vi "resetKeithley.vi"   [LabVIEW 2011, in "run.lvlib"]
uses:
  run.lvlib
  <instrlib>/Keithley 2600 Series/Keithley 2600 Series.lvlib
types:
  T1 = enum16{"Digital I/O", "TSP-Link", "LAN", "Blender", "Timer"}
  T2 = enum16{"Digital I/O", "TSP-Link", "LAN", "Blender", "Timer"}[]
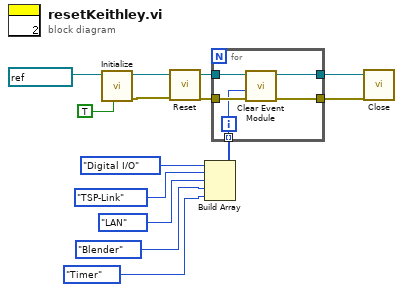
[diagram p0: block diagram]
diagram:
  n1 = call <instrlib>:"Initialize.vi"("Reset (True)"=TRUE, "VISA resource name"=refnum<visa-resource-name> "k2602a") -> ("error out"=w11:errorcluster, "VISA resource name out"=w12:refnum<visa-resource-name>)  [unwired: 8 in]
  n2 = call <instrlib>:"Reset.vi"("error in (no error)"=w11, "VISA resource name"=w12) -> ("error out"=w3:errorcluster, "VISA resource name out"=w5:refnum<visa-resource-name>)  [unwired: 8 in]
  n3 = Build Array(T1."Digital I/O" ("Event Module Type (Digital I/O)"), T1."TSP-Link" ("Event Module Type (Digital I/O)"), T1."LAN" ("Event Module Type (Digital I/O)"), T1."Blender" ("Event Module Type (Digital I/O)"), T1."Timer" ("Event Module Type (Digital I/O)")) -> (w1:T2)
  n4 = for {
    tunnel: w5 -> [w19]
    tunnel: [w18] -> w4
    tunnel: w3 -> [w17]
    tunnel: [w16] -> w2
    tunnel: w1 -> [w15] mode=indexing
    n5 = call <instrlib>:"Clear Event Module.vi"("error in"=w17, "Event Module Type (Digital I/O)"=w15, "VISA resource name"=w19) -> ("error out"=w16:errorcluster, "VISA resource name out"=w18:refnum<visa-resource-name>)  [unwired: 5 in, 2 out]
  }
  n6 = call <instrlib>:"Close.vi"("error in (no error)"=w2, "VISA resource name"=w4) -> ()  [unwired: 10 out]
